vi "Initialize.vi"(6 "FIFO Options":T10, 7 "id":i32, 8 "error in (no error)":errorcluster, 9 "Plugin Buffers":refnum<class "Buffers.lvclass">, 10 "component objects":refnum<class>[](array[class]), 11 "Plugin Configuration":T1={"name"="", "components"=[], "cycle timing"={"priority"=0, "decimation"=1, "offset"=0}, "Transfer Groups"=[], "thread count"=0, "buffer converter settings"=[], "transceiver settings"=[]} {"Transfer Groups"."Transfers"."channels"."dst buffer offset" format="%d bytes"; "Transfer Groups"."Transfers"."channels"."src buffer offset" format="%d bytes"}) -> (0 "error out":errorcluster, 2 "Plugin Threads":refnum<class "Plugin Thread.lvclass">[](array[class]), 3 "Plugin out":refnum<class "Plugin.lvclass">)   [LabVIEW 2017, in "DSF Core.lvlib" / "Plugin.lvclass"]
uses:
  Plugin.lvclass
  Typedefs/FIFO Flags.ctl
  DSF Configuration API/Public/Controls/DSF Engine Plugin Configuration.ctl
  DSF Configuration API/Public/Controls/DSF Timing Info.ctl
  DSF Configuration API/Public/Controls/DSF Engine Transfer Group Configuration.ctl
  DSF Configuration API/Public/Controls/DSF Direction.ctl
  DSF Configuration API/Public/Controls/DSF Engine Transfer Configuration.ctl
  DSF Configuration API/Public/Controls/DSF Byte Order.ctl
  DSF Configuration API/Public/Controls/DSF Engine Channel Configuration.ctl
  DSF Configuration API/Public/Controls/DSF Data Type.ctl
  DSF Configuration API/Public/Controls/DSF Settings Info.ctl
  Buffer/Buffers.lvclass
  Thread/Plugin/Plugin Thread.lvclass
  Plugin.lvclass/Plugin.ctl
  Timing/Timing.lvclass
  DSF Core.lvlib
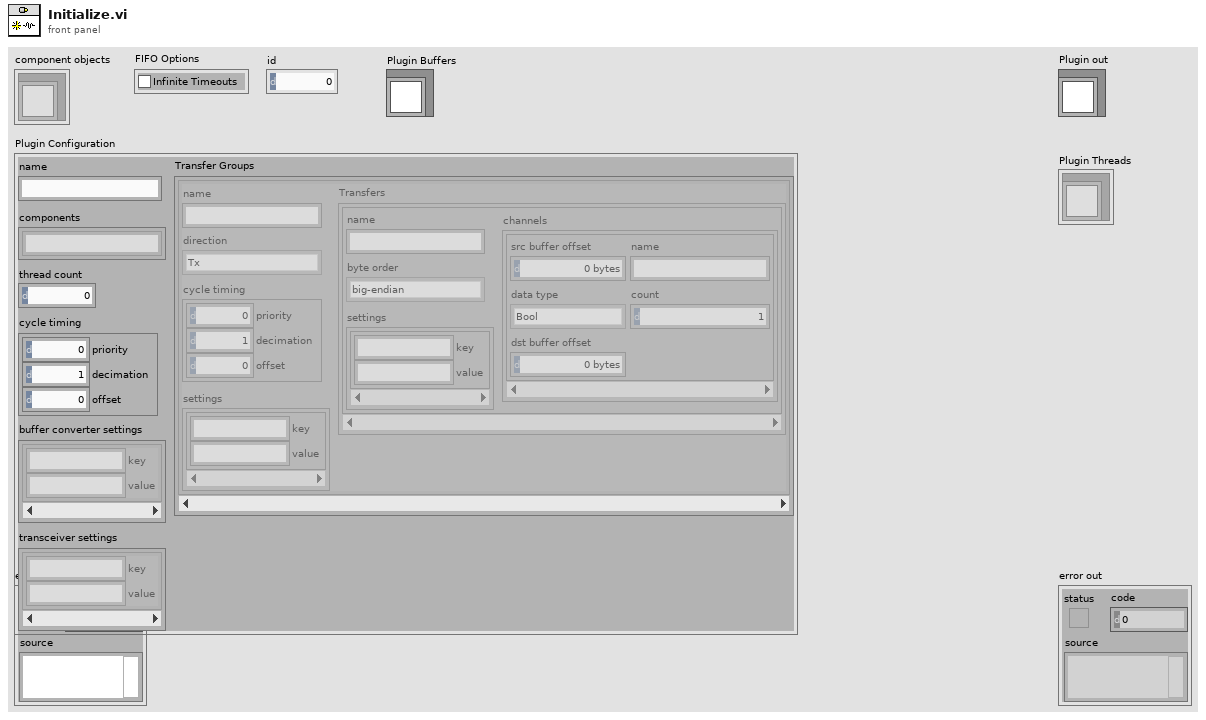
[diagram p1: front panel]
types:
  T1 = typedef "DSF Core.lvlib/DSF Engine Plugin Configuration.ctl" = cluster{"name":string, "components":string[], "cycle timing":T2, "Transfer Groups":T3[], "thread count":i32, "buffer converter settings":T9, "transceiver settings":T9}
  T2 = typedef "DSF Core.lvlib/DSF Timing Info.ctl" = cluster{"priority":u64, "decimation":u64, "offset":u64}
  T3 = typedef "DSF Core.lvlib/DSF Engine Transfer Group Configuration.ctl" = cluster{"name":string, "direction":T4, "cycle timing":T2, "Transfers":T5[], "settings":T9}
  T4 = typedef "DSF Core.lvlib/DSF Direction.ctl" = enum8{"Tx", "Rx"}
  T5 = typedef "DSF Core.lvlib/DSF Engine Transfer Configuration.ctl" = cluster{"name":string, "byte order":T6, "channels":T7[], "settings":T9}
  T6 = typedef "DSF Core.lvlib/DSF Byte Order.ctl" = enum8{"big-endian", "little-endian"}
  T7 = typedef "DSF Core.lvlib/DSF Engine Channel Configuration.ctl" = cluster{"src buffer offset":u64, "name":string, "data type":T8, "count":u64, "dst buffer offset":u64}
  T8 = typedef "DSF Core.lvlib/DSF Data Type.ctl" = enum8{"Bool", "SGL", "DBL", "I8", "I16", "I32", "I64", "U8", "U16", "U32", "U64"}
  T9 = typedef "DSF Core.lvlib/DSF Settings Info.ctl" = cluster{"key":string, "value":string}[]
  T10 = typedef "DSF Core.lvlib/FIFO Flags.ctl" = cluster{"Infinite Timeouts":bool}
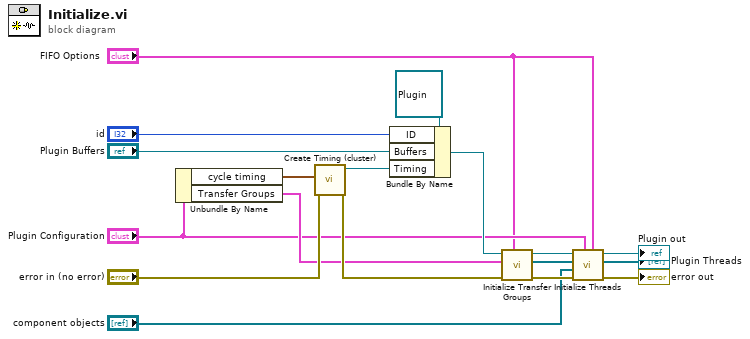
[diagram p0: block diagram]
diagram:
  n1 = Unbundle By Name("Plugin Configuration") -> ("cycle timing"=w15:T2, "Transfer Groups"=w5:T3[])
  n2 = call "Create Timing (cluster).vi"("error in (no error)"="error in (no error)", "cycle timing"=w15) -> ("error out"=w13:errorcluster, "Timing"=w8:refnum<class "Timing.lvclass">)  [unwired: 8 in]
  n3 = Bundle By Name(cluster=refnum<class "Plugin.lvclass"> refnum ("DSF Core.lvlib:Plugin"), "ID"="id", "Buffers"="Plugin Buffers", "Timing"=w8) -> (w12:refnum<class "Plugin.lvclass">)
  n4 = call "Initialize Transfer Groups.vi"("FIFO Options"="FIFO Options", "error in (no error)"=w13, "Transfer Group configurations"=w5, "Plugin in"=w12) -> ("error out"=w9:errorcluster, "Transfer Groups"=w2:refnum<class "Transfer Group.lvclass">[], "Plugin out"=w11:refnum<class "Plugin.lvclass">)  [unwired: 5 in]
  n5 = call "Initialize Threads.vi"("FIFO Options"="FIFO Options", "plugin configuration"="Plugin Configuration", "error in (no error)"=w9, "component objects"="component objects", "Transfer Groups"=w2, "Plugin in"=w11) -> ("error out"=→"error out":errorcluster, "Plugin Threads"=→"Plugin Threads":refnum<class "Plugin Thread.lvclass">[], "Plugin out"=→"Plugin out":refnum<class "Plugin.lvclass">)  [unwired: 3 in]
